vi "SubVI Tester.vi"() -> ()   [LabVIEW 2015]
uses:
  Weather Data.ctl
panel:
  in  "Weather Data":T1={"Min Temperature"=0.0, "Max Temperature"=0.0, "Current Temperature"=0.0, "Warning Text"="No Warning", "Warning?"=FALSE, "Units"=0} {"Units" items=["Fahrenheit", "Celsius"]}
  out "Weather Data Out":T1={"Min Temperature"=0.0, "Max Temperature"=0.0, "Current Temperature"=0.0, "Warning Text"="No Warning", "Warning?"=FALSE, "Units"=0} {"Units" items=["Fahrenheit", "Celsius"]}
  in  "Min Temperature":dbl=10.0
  in  "Max Temperature":dbl=30.0
  in  "Stop":bool
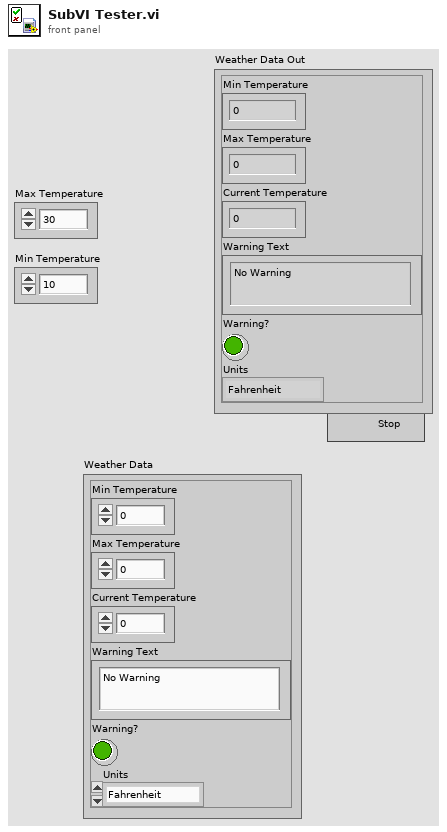
[diagram p1: front panel]
types:
  T1 = typedef "Weather Data.ctl" = cluster{"Min Temperature":dbl, "Max Temperature":dbl, "Current Temperature":dbl, "Warning Text":string, "Warning?":bool, "Units":u16}
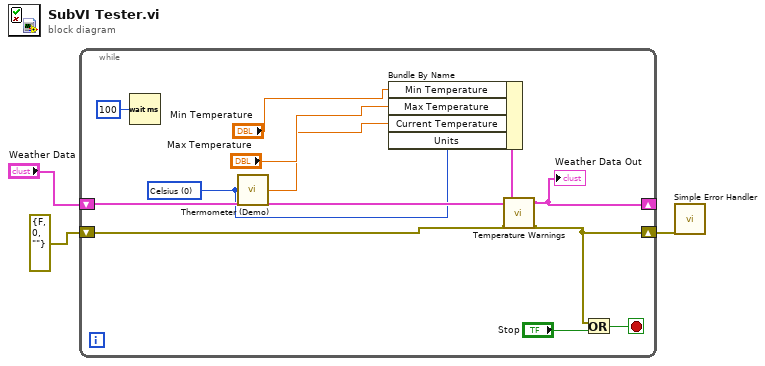
[diagram p0: block diagram]
diagram:
  n1 = while {
    shift-right: [w11] -> w3
    shift-left: errorcluster {"status"=FALSE, "code"=0, "source"=""} ("error out") -> [w10]
    shift-right: [w9] -> _
    shift-left: "Weather Data" -> [w8]
    stop <- w12 stop-if-true
    w4 = u16 0 items=["Celsius", "Fahrenheit"] ("Units (0: Celsius)")
    n2 = Wait (ms)(milliseconds to wait=u32 100) -> ()  [unwired: 1 out]
    n3 = call "Thermometer (Demo).vi"("Units (0: Celsius)"=w4) -> ("Temperature Value"=w5:dbl)
    n4 = Bundle By Name(cluster=w8, "Min Temperature"="Min Temperature", "Max Temperature"="Max Temperature", "Current Temperature"=w5, "Units"=w4) -> ()  [unwired: 1 out]
    n5 = call "Temperature Warnings.vi"("Error In"=w10, "Weather Data"=w8) -> ("Error Out"=w11:errorcluster, "Weather Data Out"=w9:T1)  [unwired: 8 in]
    "Weather Data Out" <- w9
    n6 = Or(x=w11, y="Stop") -> (x .or. y?=w12:bool)
  }
  n7 = call <vilib>:"Simple Error Handler.vi"("error in (no error)"=w3) -> ()  [unwired: 4 in, 5 out]
